vi "getStatus.vi"(8 "error in (no error)":errorcluster, 10 "AlCS in":refnum<class "AlCS.lvclass">, 11 "Heartbeat in":refnum<class "Heartbeat.lvclass">) -> (0 "error out":errorcluster, 1 "answer":string, 2 "AlCS out":refnum<class "AlCS.lvclass">, 3 "Heartbeat out":refnum<class "Heartbeat.lvclass">, 4 "newValue":bool)   [LabVIEW 2016, in "Heartbeat.lvclass"]
uses:
  Heartbeat.lvclass
  AlCS/AlCS.lvclass
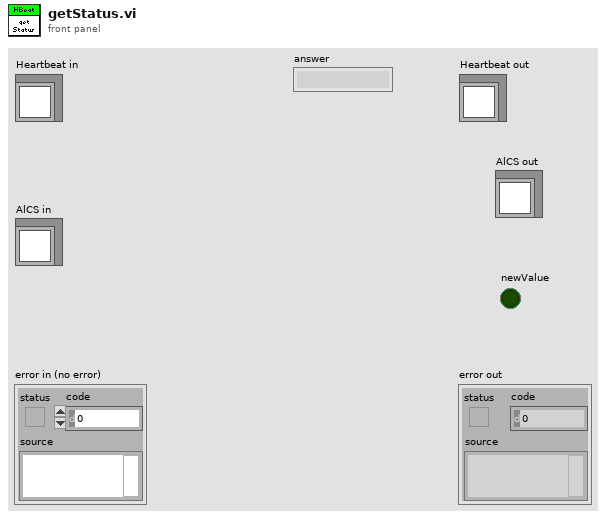
[diagram p1: front panel]
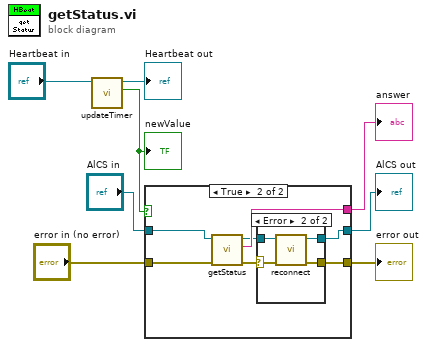
[diagram p0: block diagram]
diagram:
  n1 = call "updateTimer.vi"("Heartbeat in"="Heartbeat in") -> ("getStatus?"=w6:bool, "Heartbeat out"=→"Heartbeat out":refnum<class "Heartbeat.lvclass">)  [unwired: 8 in, 1 out]
  "newValue" <- w6
  n2 = case shown="True" w6 {
    tunnel: [w9 w13] -> w2
    tunnel: "AlCS in" -> [w10 w12]
    tunnel: [w10 w14] -> w4
    tunnel: "error in (no error)" -> [w9 w11]
    tunnel: [_ w17] -> w1
    frame False {
    }
    frame True {
      n3 = call "getStatus.vi"("error in (no error)"=w11, "AlCS in"=w12) -> ("error out"=w15:errorcluster, "answer"=w17:string, "AlCS out"=w16:refnum<class "AlCS.lvclass">)  [unwired: 7 in]
      n4 = case shown="Error" w15 {
        selector: w15 -> [w18 w22]
        tunnel: [w18 w23] -> w13
        tunnel: w16 -> [w19 w21]
        tunnel: [w19 w20] -> w14
        frame No Error {
        }
        frame Error {
          n5 = call "reconnect.vi"("error in (no error)"=w22, "AlCS in"=w21) -> ("error out"=w23:errorcluster, "AlCS out"=w20:refnum<class "AlCS.lvclass">)  [unwired: 8 in]
        }
      }
    }
  }
  "error out" <- w2
  "AlCS out" <- w4
  "answer" <- w1
